vi "Parse OM.vi"(8 "error in (no error)":errorcluster, 11 "OM in":string) -> (0 "error out":errorcluster, 3 "BML OM":T1)   [LabVIEW 2018, in "Config Parser BML.lvlib" / "Config Parser BML.lvclass"]
uses:
  Config Parser BML.lvclass
  Ctls/OM - BML.ctl
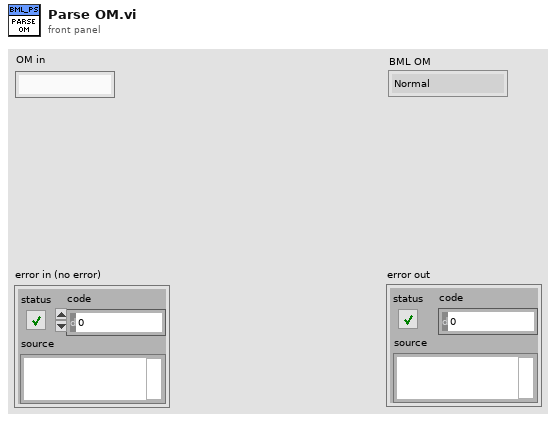
[diagram p1: front panel]
types:
  T1 = typedef "OM - BML.ctl" = enum16{"Normal", "ImmeEffect", "InitSlaveID", "LoadData"}
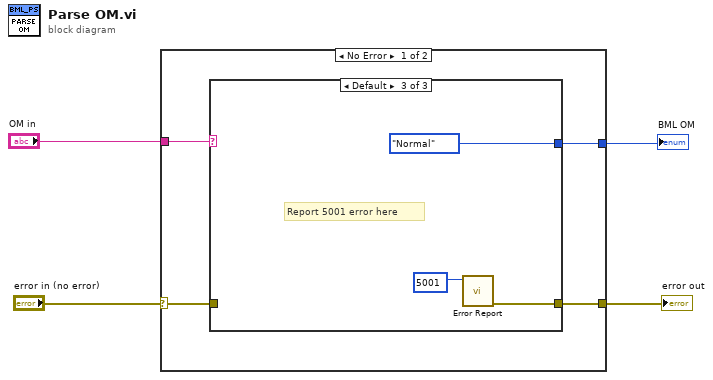
[diagram p0: block diagram]
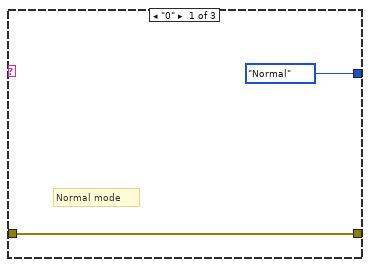
[diagram p2: hidden frame]
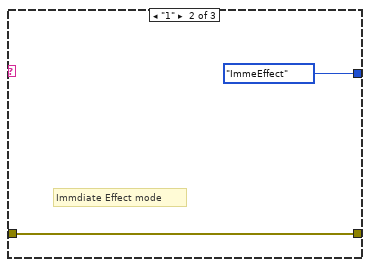
[diagram p3: hidden frame]
diagram:
  n1 = case shown="No Error" "error in (no error)" {
    selector: "error in (no error)" -> [w8 w16]
    tunnel: "OM in" -> [w7 _]
    tunnel: [w6 w16] -> w2
    tunnel: [w5 _] -> w1
    frame No Error {
      n2 = case shown="Default" w7 {
        tunnel: w8 -> [w10 w12 _]
        tunnel: [w10 w12 w14] -> w6
        tunnel: [OM_-_BML."Normal" ("BML OM") OM_-_BML."ImmeEffect" ("BML OM") OM_-_BML."Normal" ("BML OM")] -> w5
        frame "0" {
          # "Normal mode"
        }
        frame "1" {
          # "Immdiate Effect mode"
        }
        frame Default {
          # "Report 5001 error here"
          n3 = call "Error Report.vi"("Error Code"=i16 5001) -> ("error out"=w14:errorcluster)  [unwired: 10 in]
        }
      }
    }
    frame Error {
    }
  }
  "error out" <- w2
  "BML OM" <- w1
